vi "Solonoid Launcher.vi"(8 "error in (no error)":errorcluster, 9 "Sub Panel":refnum<vi>, 10 "Solenoid ID":string="Secondary", 11 "Feeder Actor In":refnum<class "Feeder.lvclass">) -> (0 "error out":errorcluster, 2 "Nested Actor's Enqueuer":refnum<class "Message Enqueuer.lvclass">, 3 "Feeder Actor Out":refnum<class "Feeder.lvclass">)   [LabVIEW 2018, in "Feeder Actor.lvlib" / "Solenoid.lvclass"]
uses:
  Solenoid.lvclass
  <vilib>/ActorFramework/Message Enqueuer/Message Enqueuer.lvclass
  Feeder/Feeder.lvclass
  C:/Program Files/National Instruments/LabVIEW 2018/vi.lib/MGI/Panel Manager/Panel Actor/Panel Actor/Panel Actor.lvclass
  Solenoid.lvclass/Solenoid.ctl
  <vilib>/DAQmx/write.llb/DAQmx Write (Digital Bool 1Line 1Point).vi
  <vilib>/MGI/Panel Manager/Panel/Panel/Subpanel/Subpanel.lvclass
  C:/Program Files/National Instruments/LabVIEW 2018/vi.lib/MGI/Panel Manager/Panel/Panel/Panel.lvclass
  <vilib>/DAQmx/create/channels.llb/DAQmx Create Channel (DO-Digital Output).vi
  <vilib>/DAQmx/miscellaneous.llb/DAQmx Fill In Error Info.vi
  <vilib>/MGI/Panel Manager/Panel/Panel/Subpanel/Subpanel.vi
  <vilib>/MGI/Panel Manager/Panel/Panel.lvlib
  <vilib>/MGI/Panel Manager/Panel Actor/Panel Actor/Panel Actor.lvclass
  ADM/Main.lvlib
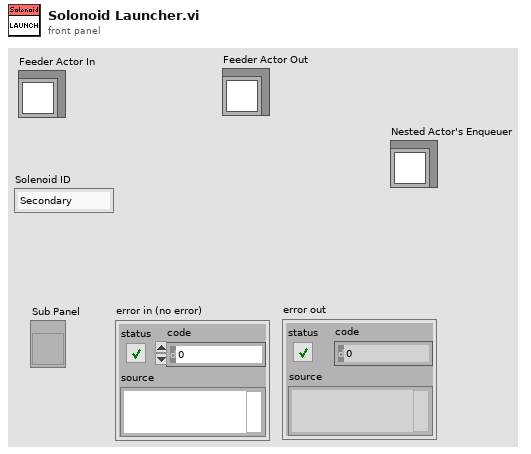
[diagram p1: front panel]
types:
  T1 = cluster{"Task Name":string, "Task Type":enum16{"VISA", "DAQmx"}, "VISA Resource Name":refnum<visa-resource-name>, "DAQmx Channel Name":tag}
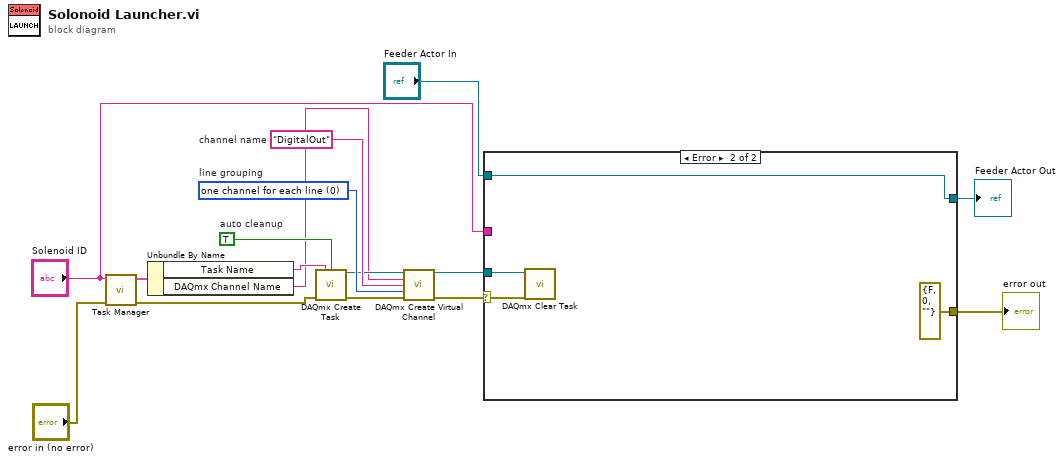
[diagram p0: block diagram]
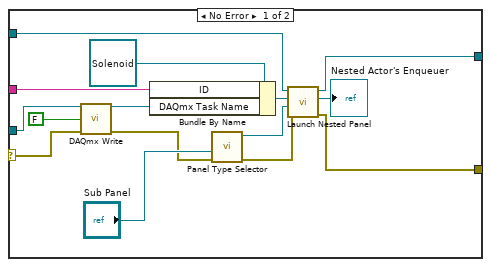
[diagram p2: hidden frame]
diagram:
  w13 = 0 items=["one channel for each line", "one channel for all lines"]  # line grouping
  w14 = "DigitalOut"  # channel name
  w11 = TRUE  # auto cleanup
  n1 = call "Task Manager.vi"("error in (no error)"="error in (no error)", "Task"="Solenoid ID") -> ("error out"=w2:errorcluster, "Task Properties"=w6:T1)  [unwired: 8 in]
  n2 = Unbundle By Name(w6) -> ("Task Name"=w5:string, "DAQmx Channel Name"=w4:tag)
  n3 = call <vilib>:"DAQmx Create Task.vi"("new task name"=w5, "auto cleanup"=w11, "error in"=w2) -> ("task out"=w12:refnum<k21>, "error out"=w10:errorcluster)  [unwired: 11 in]
  n4 = call-poly <vilib>:"DAQmx Create Virtual Channel.vi"("task in"=w12, "lines"=w4, "name to assign"=w14, "line grouping"=w13, "error in"=w10) -> ("task out"=w8:refnum<k21>, "error out"=w9:errorcluster)  [unwired: 9 in]
  n5 = case shown="Error" w9 {
    selector: w9 -> [w20 w33]
    tunnel: "Feeder Actor In" -> [w26 w35]
    tunnel: [w25 w35] -> w15
    tunnel: "Solenoid ID" -> [w24 _]
    tunnel: w8 -> [w23 w34]
    tunnel: [w17 errorcluster {"status"=FALSE, "code"=0, "source"=""} ("error out")] -> w1
    frame No Error {
      n6 = call-poly <vilib>:"DAQmx Write.vi"("task/channels in"=w23, "data"=FALSE, "error in"=w20) -> ("task out"=w22:refnum<k21>, "error out"=w19:errorcluster)  [unwired: 10 in, 1 out]
      n7 = Bundle By Name(cluster=refnum<class "Solenoid.lvclass"> refnum ("Feeder Actor.lvlib:Solenoid.lvclass"), "ID"=w24, "DAQmx Task Name"=w22) -> (w28:refnum<class "Solenoid.lvclass">)
      n8 = call-poly <vilib>:"Panel Type Selector.vi"("Error In"=w19, "Sub Panel"="Sub Panel") -> ("Error Out"=w18:errorcluster, "Subpanel Out"=w29:refnum<class "Subpanel.lvclass">)  [unwired: 8 in]
      n9 = call <vilib>:"Launch Nested Panel.vi"("error in (no error)"=w18, "Panel"=w29, "Nested Panel Actor"=w28, "Panel Actor in"=w26) -> ("error out"=w17:errorcluster, "Nested Actor's Enqueuer"=→"Nested Actor's Enqueuer":refnum<class "Message Enqueuer.lvclass">, "Panel Actor out"=w25:refnum<class "Feeder.lvclass">)  [unwired: 4 in, 1 out]
    }
    frame Error {
      n10 = call <vilib>:"DAQmx Clear Task.vi"("task in"=w34, "error in"=w33) -> ()  [unwired: 13 in, 1 out]
    }
  }
  "Feeder Actor Out" <- w15
  "error out" <- w1
